vi "read station ethernet config.vi"(8 "error in":errorcluster, 10 "station idx":i32, 11 "configuration file path in":path) -> (0 "error out":errorcluster, 2 "ethernet address map":T1, 3 "configuration file path out":path)   [LabVIEW 2018]
uses:
  02.Type Def's/station ethernet address map.ctl
  05.UserVI's/file io/ini/type defs/ini file actions.ctl
  05.UserVI's/file io/ini/type defs/ini entry value.ctl
  05.UserVI's/file io/ini/type defs/ini entry types.ctl
  05.UserVI's/file io/ini/type defs/ini entry.ctl
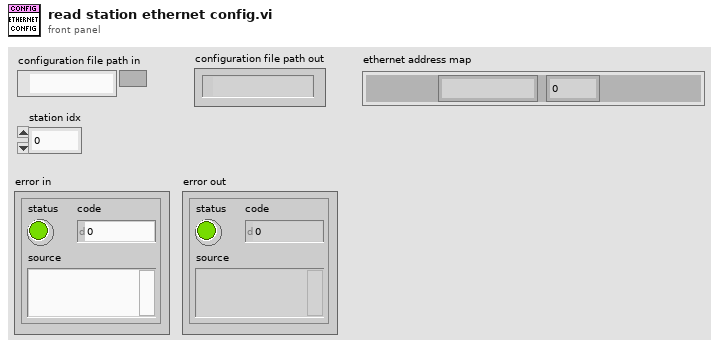
[diagram p1: front panel]
types:
  T1 = typedef "station ethernet address map.ctl" = cluster{"LVDT 1 Unit":string, "LVDT Unit 1 port":u16}
  T2 = typedef "ini entry value.ctl" = cluster{"Boolean":bool, "Dbl":dbl, "I32":i32, "Path":path, "String":string, "U32":u32}
  T3 = typedef "ini file actions.ctl" = enum16{"read ini", "write ini"}
  T4 = typedef "ini entry.ctl" = cluster{"section":string, "key":string, "type":T5, "default value":T2}
  T5 = typedef "ini entry types.ctl" = enum16{"Boolean", "Double", "I32", "Path", "String", "U32"}
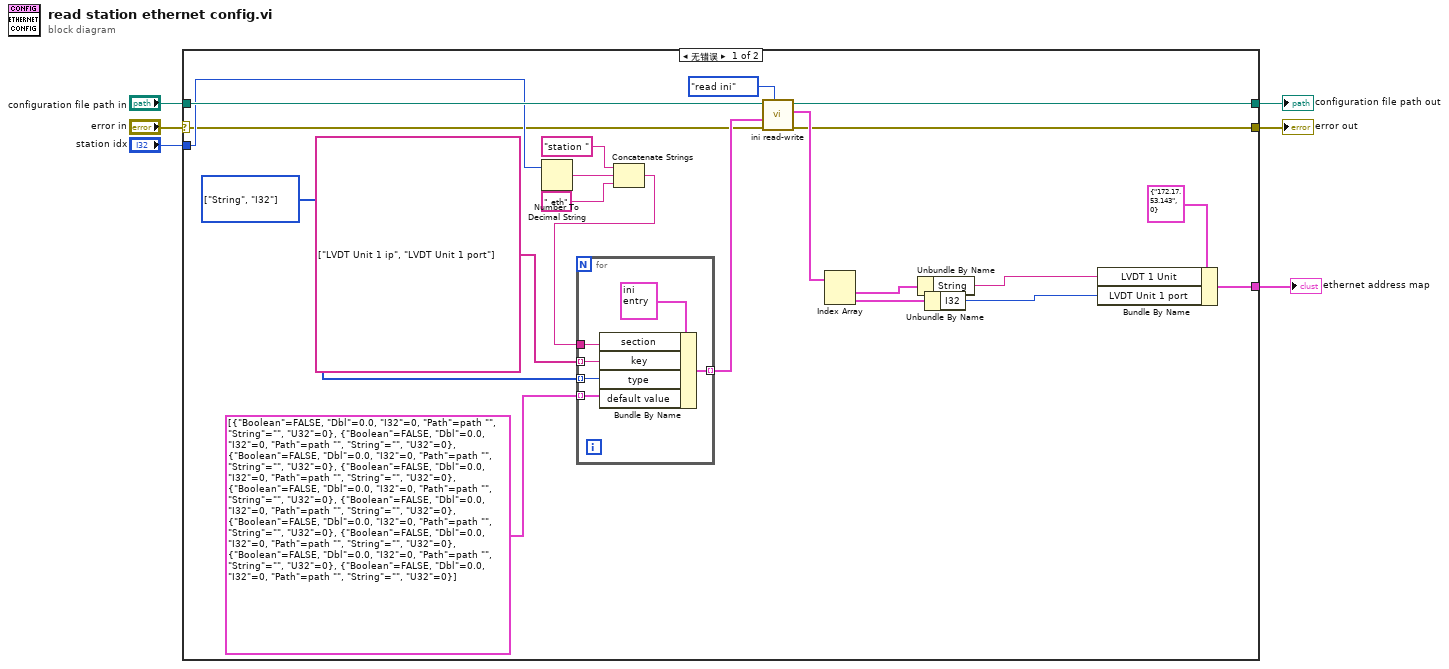
[diagram p0: block diagram]
diagram:
  n1 = case shown="无错误" "error in" {
    selector: "error in" -> [w13 w35]
    tunnel: [w27 _] -> w1
    tunnel: "configuration file path in" -> [w26 w34]
    tunnel: [w23 w34] -> w5
    tunnel: [w22 w35] -> w4
    tunnel: "station idx" -> [w20 _]
    frame No Error {
      w16 = T5[] [enum."String", enum."I32"] items=["Boolean", "Double", "I32", "Path", "String", "U32"]
      n2 = Number To Decimal String(number=w20) -> (decimal integer string=w19:string)  [unwired: 1 in]
      n3 = Concatenate Strings("station ", w19, " eth" ("string")) -> (w18:string)
      n4 = for {
        tunnel: w18 -> [w32]
        tunnel: string[] ["LVDT Unit 1 ip", "LVDT Unit 1 port"] -> [w31] mode=indexing
        tunnel: w16 -> [w30] mode=indexing
        tunnel: T2[] [{"Boolean"=FALSE, "Dbl"=0.0, "I32"=0, "Path"=path "", "String"="", "U32"=0}, {"Boolean"=FALSE, "Dbl"=0.0, "I32"=0, "Path"=path "", "String"="", "U32"=0}, {"Boolean"=FALSE, "Dbl"=0.0, "I32"=0, "Path"=path "", "String"="", "U32"=0}, {"Boolean"=FALSE, "Dbl"=0.0, "I32"=0, "Path"=path "", "String"="", "U32"=0}, {"Boolean"=FALSE, "Dbl"=0.0, "I32"=0, "Path"=path "", "String"="", "U32"=0}, {"Boolean"=FALSE, "Dbl"=0.0, "I32"=0, "Path"=path "", "String"="", "U32"=0}, {"Boolean"=FALSE, "Dbl"=0.0, "I32"=0, "Path"=path "", "String"="", "U32"=0}, {"Boolean"=FALSE, "Dbl"=0.0, "I32"=0, "Path"=path "", "String"="", "U32"=0}, {"Boolean"=FALSE, "Dbl"=0.0, "I32"=0, "Path"=path "", "String"="", "U32"=0}, {"Boolean"=FALSE, "Dbl"=0.0, "I32"=0, "Path"=path "", "String"="", "U32"=0}] -> [w29] mode=indexing
        tunnel: [w28] -> w14 mode=indexing
        n5 = Bundle By Name(cluster=T4 {"section"="", "key"="", "type"=enum."Boolean", "default value"={"Boolean"=FALSE, "Dbl"=0.0, "I32"=0, "Path"=path "", "String"="", "U32"=0}}, "section"=w32, "key"=w31, "type"=w30, "default value"=w29) -> (w28:T4)
      }
      n6 = call "ini read-write.vi"("action"=ini_file_actions."read ini", "error in (no error)"=w13, "ini entry descriptors"=w14, "configuration file path"=w26) -> ("error out"=w22:errorcluster, "values out"=w24:T2[], "configuration file path out"=w23:path)  [unwired: 5 in]
      n7 = Index Array(array=w24) -> (element #1=w9:T2, element #2=w10:T2)  [unwired: 2 in]
      n8 = Unbundle By Name(w9) -> ("String"=w8:string)
      n9 = Unbundle By Name(w10) -> ("I32"=w7:i32)
      n10 = Bundle By Name(cluster=T1 {"LVDT 1 Unit"="172.17.53.143", "LVDT Unit 1 port"=0} ("ethernet address map"), "LVDT 1 Unit"=w8, "LVDT Unit 1 port"=w7) -> (w27:T1)
    }
    frame Error {
    }
  }
  "configuration file path out" <- w5
  "error out" <- w4
  "ethernet address map" <- w1
